vi "Init Hardware.vi"(8 "error in (no error)":errorcluster, 11 "DAQmx Digitizer in":refnum<class "DAQmx Digitizer.lvclass">) -> (0 "error out":errorcluster, 3 "DAQmx Digitizer out":refnum<class "DAQmx Digitizer.lvclass">)   [LabVIEW 2015, in "DAQmx Digitizer.lvclass"]
uses:
  DAQmx Digitizer.lvclass
  Instruments/Pulse Driver/Pulse Driver.lvclass/Pulse Driver.ctl
  DAQmx Digitizer.lvclass/DAQmx Digitizer.ctl
  Instruments/Pulse Driver/Read User Configuration.vi
  Instruments/Pulse Driver/Read Pretrigger samples.vi
  Instruments/Pulse Driver/Read Samples per channel.vi
  Instruments/Pulse Driver/Write Scaling coefficients.vi
  Instruments/Pulse Driver/Write Channel names.vi
  Instruments/Pulse Driver/Write User Configuration.vi
  <vilib>/DAQmx/create/channels.llb/DAQmx Create Channel (AI-Voltage-Basic).vi
  <vilib>/DAQmx/configure/timing.llb/DAQmx Timing (Sample Clock).vi
  <vilib>/DAQmx/configure/trigger.llb/DAQmx Reference Trigger (Digital Edge).vi
  <resource>/objmgr/daqmx.rc
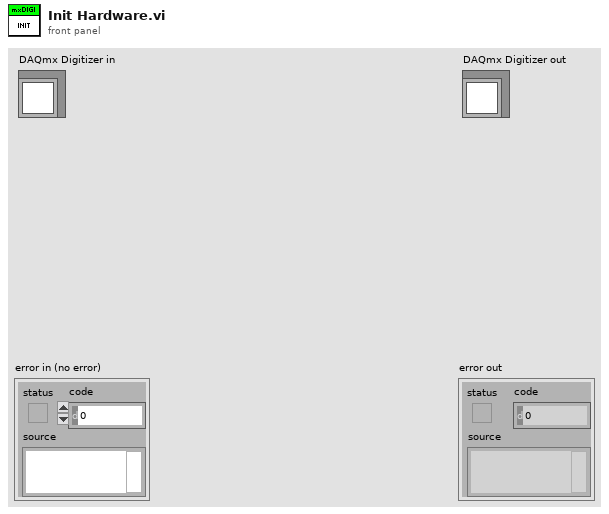
[diagram p1: front panel]
types:
  T1 = typedef "Pusle Driver Configuration.ctl" = cluster{"Pre-trigger duration":dbl, "Post-trigger duration":dbl, "Rate":dbl, "Ranges":dbl[], "Re-name channels":string[], "Active channels":string, "External clock":bool}
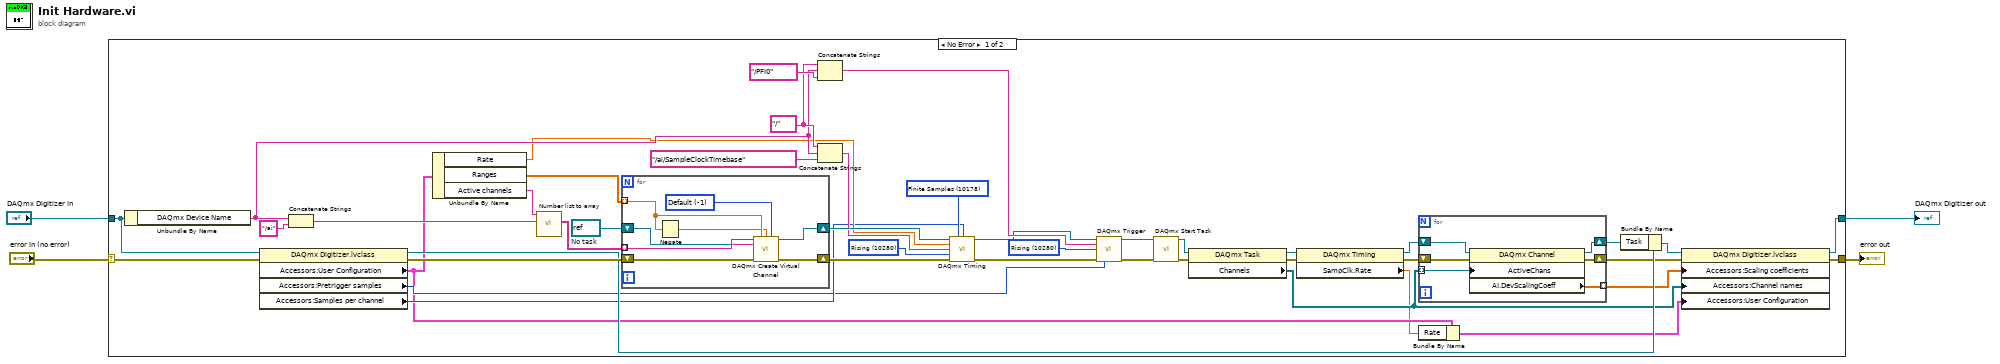
[diagram p0: block diagram]
diagram:
  n1 = case shown="No Error" "error in (no error)" {
    selector: "error in (no error)" -> [w22 w64]
    tunnel: [w23 w64] -> w3
    tunnel: [w24 w63] -> w1
    tunnel: "DAQmx Digitizer in" -> [w20 w63]
    frame No Error {
      w27 = refnum<k21> refnum  # No task
      w35 = 10280 items=["Rising"=10280, "Falling"=10171] ("active edge")
      w36 = 10178 items=["Finite Samples"=10178, "Continuous Samples"=10123, "Hardware Timed Single Point"=12522] ("sample mode")
      w38 = tag "/" ("string")
      w46 = 10280 items=["Rising"=10280, "Falling"=10171] ("edge")
      n2 = Unbundle By Name(w20) -> ("DAQmx Device Name"=w28:tag)
      n3 = property class="DAQmx Digitizer.lvclass"(reference=w20, error in=w22) -> (reference out=w19:refnum<class "DAQmx Digitizer.lvclass">, error out=w21:errorcluster, "Accessors:User Configuration"=w8:T1, "Accessors:Pretrigger samples"=w9:u32, "Accessors:Samples per channel"=w10:i32)
      n4 = Concatenate Strings(w28, "/ai" ("string")) -> (w29:string)
      n5 = Unbundle By Name(w8) -> ("Rate"=w25:dbl, "Ranges"=w5:dbl[], "Active channels"=w31:string)
      n6 = call "Number list to array.vi"("Full names prefix"=w29, "Number list"=w31) -> ("Full names"=w26:string[])  [unwired: 8 in, 1 out]
      n7 = for {
        tunnel: w26 -> [w62] mode=indexing
        tunnel: w5 -> [w60] mode=indexing
        shift-right: [w57] -> w45
        shift-left: w21 -> [w61]
        shift-right: [w58] -> w48
        shift-left: w27 -> [w55]
        w56 = -1 items=["Default"=-1, "RSE"=10083, "NRSE"=10078, "Differential"=10106, "Pseudodifferential"=12529] ("input terminal configuration")
        n8 = Negate(x=w60) -> (-x=w59:dbl)
        n9 = call-poly <vilib>:"DAQmx Create Virtual Channel.vi"("task in"=w55, "maximum value"=w60, "minimum value"=w59, "input terminal configuration"=w56, "physical channels"=w62, "error in"=w61) -> ("task out"=w58:refnum<k21>, "error out"=w57:errorcluster)  [unwired: 8 in]
      }
      n10 = Concatenate Strings(w38, w28, tag "/PFI0" ("string")) -> (w41:string)
      n11 = Concatenate Strings(w38, w28, tag "/ai/SampleClockTimebase" ("string")) -> (w34:string)
      n12 = call-poly <vilib>:"DAQmx Timing.vi"("task/channels in"=w48, "sample mode"=w36, "samples per channel"=w10, "rate"=w25, "source"=w34, "active edge"=w35, "error in"=w45) -> ("task out"=w39:refnum<k21>, "error out"=w40:errorcluster)  [unwired: 7 out]
      n13 = call-poly <vilib>:"DAQmx Trigger.vi"("task/channels in"=w39, "source"=w41, "edge"=w46, "error in"=w40, "pretrigger samples per channel"=w9) -> ("task out"=w42:refnum<k21>, "error out"=w43:errorcluster)  [unwired: 9 out]
      n14 = call <vilib>:"DAQmx Start Task.vi"("task/channels in"=w42, "error in"=w43) -> ("task out"=w33:refnum<k21>, "error out"=w32:errorcluster)  [unwired: 12 out]
      n15 = property class="DAQmx Task"(reference=w33, error in=w32) -> (reference out=w18:refnum<k21>, error out=w17:errorcluster, "Channels"=w16:refnum<k21>[])
      n16 = property class="DAQmx Timing"(reference=w18, error in=w17) -> (reference out=w14:refnum<k21>, error out=w15:errorcluster, "SampClk.Rate"=w7:dbl)
      n17 = for {
        tunnel: w16 -> [w54] mode=indexing
        shift-right: [w51] -> w13
        shift-left: w14 -> [w52]
        shift-right: [w50] -> w12
        shift-left: w15 -> [w53]
        tunnel: [w49] -> w11 mode=indexing
        n18 = property class="DAQmx Channel"(reference=w52, error in=w53, "ActiveChans"=w54) -> (reference out=w51:refnum<k21>, error out=w50:errorcluster, "AI.DevScalingCoeff"=w49:dbl[])
      }
      n19 = Bundle By Name(cluster=w8, "Rate"=w7) -> (w6:T1)
      n20 = Bundle By Name(cluster=w19, "Task"=w13) -> (w44:refnum<class "DAQmx Digitizer.lvclass">)
      n21 = property class="DAQmx Digitizer.lvclass"(reference=w44, error in=w12, "Accessors:Scaling coefficients"=w11, "Accessors:Channel names"=w16, "Accessors:User Configuration"=w6) -> (reference out=w24:refnum<class "DAQmx Digitizer.lvclass">, error out=w23:errorcluster)
    }
    frame Error {
    }
  }
  "error out" <- w3
  "DAQmx Digitizer out" <- w1
